vi "Init.vi"(8 "error in (no error)":errorcluster, 10 "Game (readonly)":refnum<class "Game.lvclass">, 11 "GameMenu in":refnum<class "GameMenu.lvclass">) -> (0 "error out":errorcluster, 3 "GameMenu out":refnum<class "GameMenu.lvclass">, 4 "CursorSprite":refnum<class "RT_Sprite.lvclass">)   [LabVIEW 2019, in "RT_Game.lvlib" / "GameMenu.lvclass"]
uses:
  GameMenu.lvclass
  RT_Sprite/RT_Sprite.lvclass
  C:/Users/FreshBob/Dropbox/VIs/myRIO_GameConsole/RT/RT_Game/GameObject/GameObject.lvclass
  Game/Game.lvclass
  GameMenu.lvclass/GameMenu.ctl
  Game/Coordinate.ctl
  GameObject/GameObject.lvclass/GameObject.ctl
  Game/Game.lvclass/Game.ctl
  GameObject/Write IsActive.vi
  Game/Read Singleplayer.vi
  GameObject/GameObject.lvclass
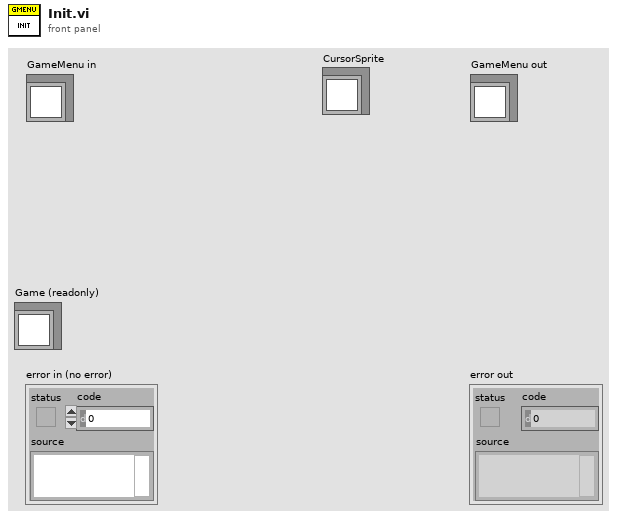
[diagram p1: front panel]
types:
  T1 = typedef "RT_Game.lvlib/Game.lvclass/Coordinate.ctl" = cluster{"x":dbl, "y":dbl}
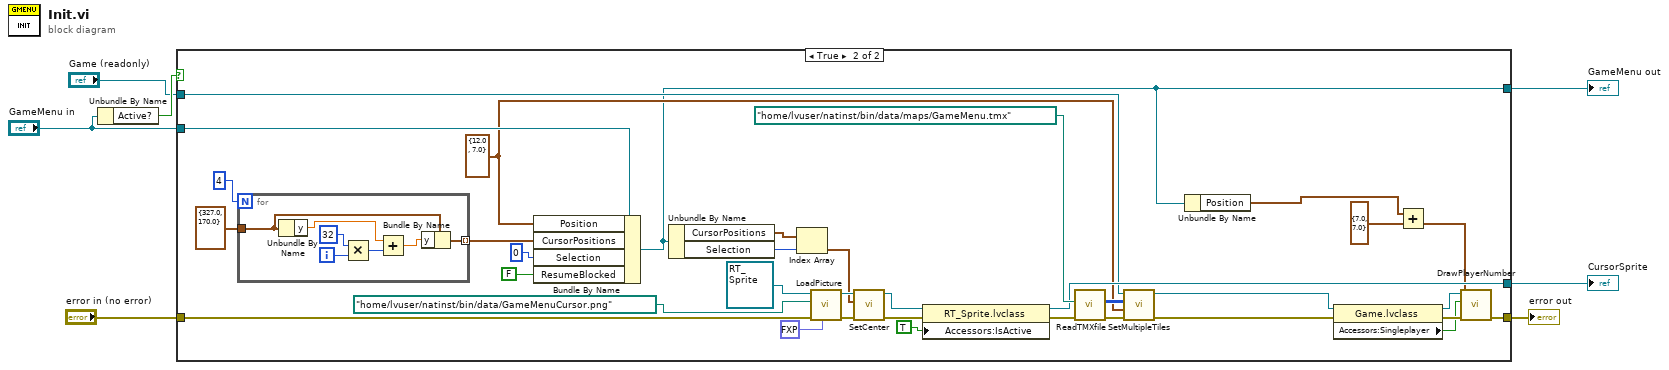
[diagram p0: block diagram]
diagram:
  n1 = Unbundle By Name("GameMenu in") -> ("Active?"=w6:bool)
  n2 = case shown="True" w6 {
    tunnel: "error in (no error)" -> [w9 w15]
    tunnel: [w9 w18] -> w5
    tunnel: "GameMenu in" -> [w8 w39]
    tunnel: [w8 w12] -> w3
    tunnel: [_ w27] -> w2
    tunnel: "Game (readonly)" -> [_ w16]
    frame False {
    }
    frame True {
      w23 = T1 {"x"=12.0, "y"=7.0} ("Position")
      n3 = for {
        N: 4 -> [_]
        tunnel: T1 {"x"=327.0, "y"=170.0} ("Position") -> [w50]
        tunnel: [w51] -> w30 mode=indexing
        i -> [w47]
        n4 = Unbundle By Name(w50) -> ("y"=w49:dbl)
        n5 = Multiply(x=32, y=w47) -> (x*y=w45:i32)
        n6 = Add(x=w49, y=w45) -> (x+y=w48:dbl)
        n7 = Bundle By Name(cluster=w50, "y"=w48) -> (w51:T1)
      }
      n8 = Bundle By Name(cluster=w39, "Position"=w23, "CursorPositions"=w30, "Selection"=i16 0, "ResumeBlocked"=FALSE ("Boolean")) -> (w12:refnum<class "GameMenu.lvclass">)
      n9 = Unbundle By Name(w12) -> ("CursorPositions"=w38:T1[], "Selection"=w37:i16)
      n10 = Index Array(array=w38, index=w37) -> (element=w33:T1)
      n11 = call "LoadPicture.vi"("Transparent Color"=fxp<+,3,3> 2.0, "error in (no error)"=w15, "Picture Path"=path "/home/lvuser/natinst/bin/data/GameMenuCursor.png", "RT_Sprite in"=refnum<class "RT_Sprite.lvclass"> refnum ("RT_Game.lvlib:RT_Sprite.lvclass")) -> ("error out"=w36:errorcluster, "RT_Sprite out"=w34:refnum<class "RT_Sprite.lvclass">)  [unwired: 6 in]
      n12 = call "SetCenter.vi"("error in (no error)"=w36, "center_position"=w33, "GameObject in"=w34) -> ("error out"=w35:errorcluster, "GameObject out"=w28:refnum<class "RT_Sprite.lvclass">)  [unwired: 7 in]
      n13 = property class="RT_Sprite.lvclass"(reference=w28, error in=w35, "Accessors:IsActive"=TRUE ("IsActive")) -> (reference out=w27:refnum<class "RT_Sprite.lvclass">, error out=w29:errorcluster)
      n14 = call "ReadTMXfile.vi"("error in (no error)"=w29, "path to tmx-file (created with Tiles2D)"=path "/home/lvuser/natinst/bin/data/maps/GameMenu.tmx") -> ("error out"=w43:errorcluster, "Tilenumbers"=w24:u32[][])  [unwired: 8 in]
      n15 = call "SetMultipleTiles.vi"("error in (no error)"=w43, "Position"=w23, "TileCodes"=w24, "Game in"=w16) -> ("error out"=w19:errorcluster, "Game out"=w17:refnum<class "Game.lvclass">)  [unwired: 6 in]
      n16 = Unbundle By Name(w12) -> ("Position"=w11:T1)
      n17 = property class="Game.lvclass"(reference=w17, error in=w19) -> (reference out=w21:refnum<class "Game.lvclass">, error out=w22:errorcluster, "Accessors:Singleplayer"=w20:bool)
      n18 = Add(x=w11, y=T1 {"x"=7.0, "y"=7.0} ("Position")) -> (x+y=w13:T1)
      n19 = call "DrawPlayerNumber.vi"("error in (no error)"=w22, "Position"=w13, "Accessors:Singleplayer"=w20, "Game in"=w21) -> ("error out"=w18:errorcluster)  [unwired: 7 in]
    }
  }
  "GameMenu out" <- w3
  "error out" <- w5
  "CursorSprite" <- w2
